vi "DeleteAProperty.vi"(7 "Position Index":T11, 8 "error IO":errorcluster, 10 "JSON Text":string, 11 "Data":T1) -> (0 "error out":errorcluster, 1 "Position Index Out":T11, 2 "JSON Text out":string, 3 "Data Out":T1)   [LabVIEW 2017]
uses:
  <vilib>/JDP Science/JSONtext/JSONtext.lvlib
  8dd03d57-00a7-4a41-af65-d2a72e3468d9.vi
  ab79f004-401f-4e0e-8bc0-55245355768b.vi
  fc2bac9e-75c4-4cb1-9ee7-1f7125c17c3a.vi
  f6ad1758-55d4-4416-b90a-648c1bc133c8.vi
  Ctrl/Property.ctl
  Ctrl/PhysicalChannel.ctl
  Ctrl/Bitfield.ctl
  Ctrl/Register.ctl
  Ctrl/ScaleType.ctl
  Ctrl/Scale.ctl
  Ctrl/EnumValue.ctl
  Ctrl/Enum.ctl
  Ctrl/Caps.ctl
  Ctrl/Data.ctl
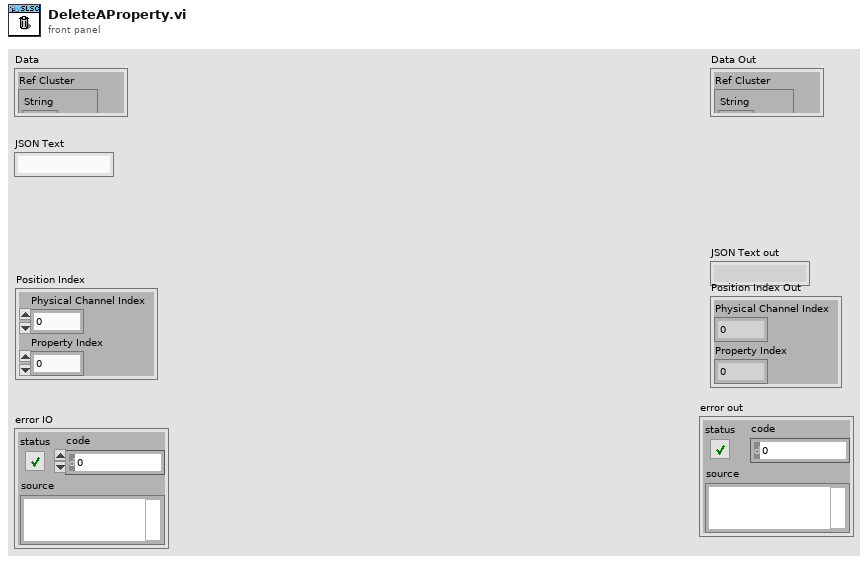
[diagram p1: front panel]
types:
  T1 = typedef "Data.ctl" = cluster{"Ref Cluster":cluster{"String":refnum<vi>, "U8":refnum<vi>, "I8":refnum<vi>, "U32":refnum<vi>, "I32":refnum<vi>, "U64":refnum<vi>, "I64":refnum<vi>, "Ring":refnum<vi>, "DBL":refnum<vi>, "Add":refnum<vi>, "Remove":refnum<vi>, "Property tree":refnum<vi>, "confirm":refnum<vi>}, "JSON Text":string, "Original JSON Text":string, "Caps":T2, "SLSC Output Tree":cluster{"Left Cell String":string, "Child Text":string[], "Child Tag":string, "Item Indent":i32, "Child Only?":bool, "Glyph Index":i32, "offline value":variant}[], "Ref Index and Control Type":cluster{"index":i32, "Datatype":string}, "Selected Type and name":cluster{"Selected Type":enum16{"Property", "Physical Channel", "Other"}, "Selected Property Name":string}, "Update whole Tree?":bool}
  T2 = typedef "Caps.ctl" = cluster{"properties":T3[], "physical channels":T4[], "registers":T5[], "scales":T7[], "enums":T9[], "productName":string}
  T3 = typedef "Property.ctl" = cluster{"name":string, "bitfield":string, "value":variant, "dataType":string, "min":variant, "max":variant, "scale":string, "access":string}
  T4 = typedef "PhysicalChannel.ctl" = cluster{"name":string, "properties":T3[]}
  T5 = typedef "Register.ctl" = cluster{"name":string, "address":i32, "size":i32, "bitfields":T6[], "initialValue":variant, "connectedProperties":string[]}
  T6 = typedef "Bitfield.ctl" = cluster{"name":string, "offset":i32, "size":i32, "signed":bool}
  T7 = typedef "Scale.ctl" = cluster{"name":string, "type":T8, "params":variant}
  T8 = typedef "ScaleType.ctl" = enum16{"NoScale", "Table", "Polynomial", "Linear"}
  T9 = typedef "Enum.ctl" = cluster{"name":string, "values":T10[]}
  T10 = typedef "EnumValue.ctl" = cluster{"name":string, "value":i32}
  T11 = cluster{"Physical Channel Index":i32, "Property Index":i32}
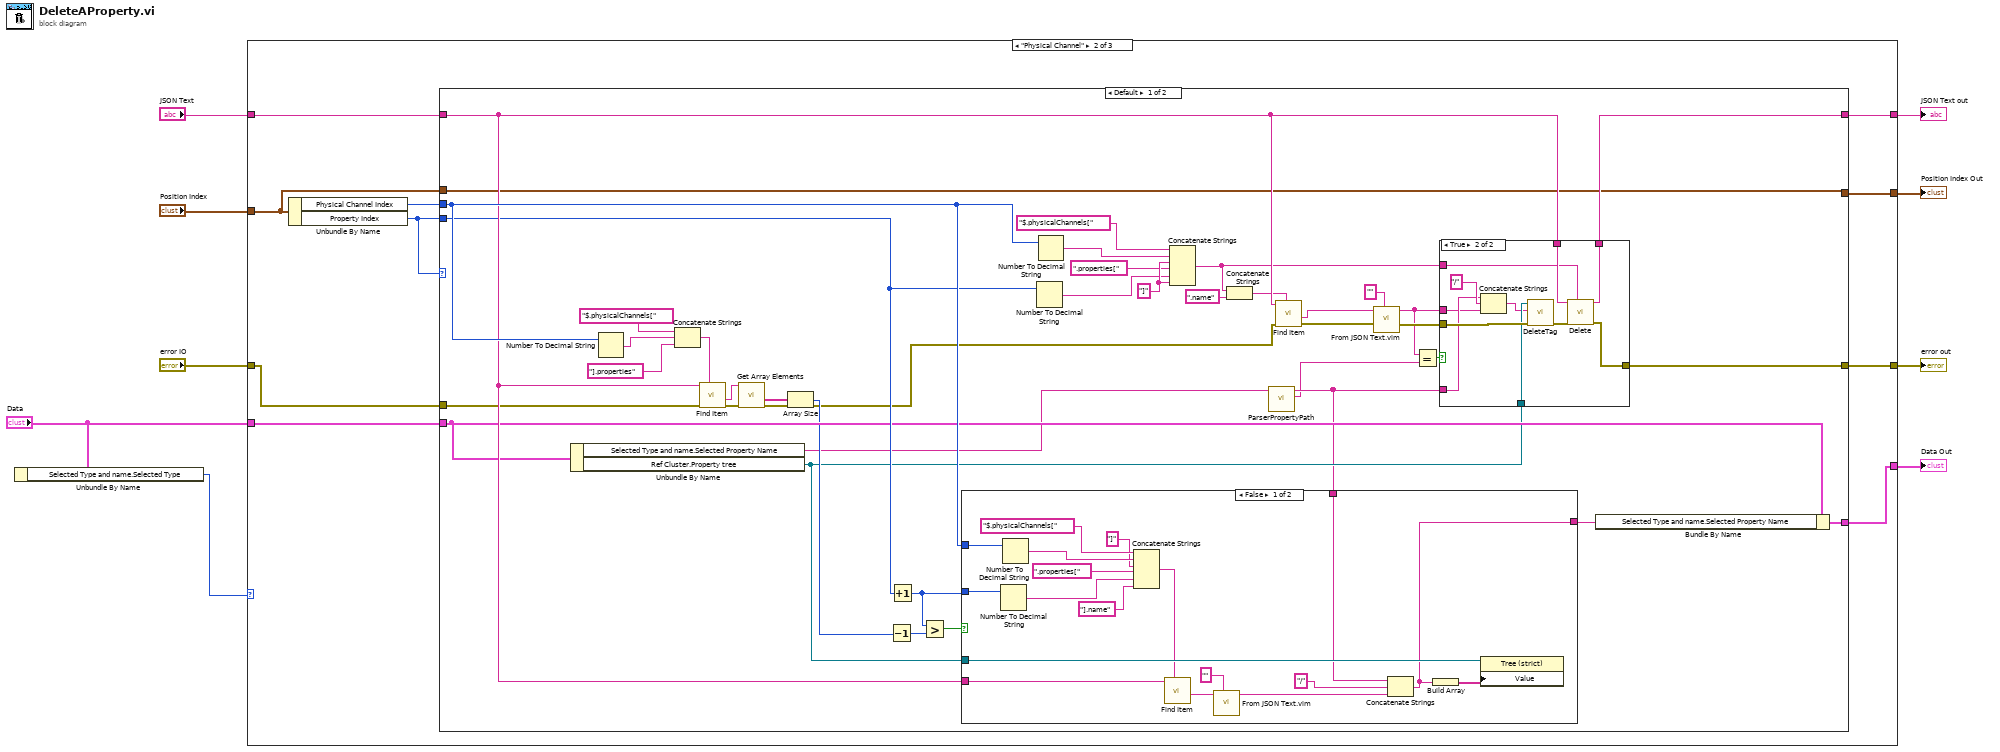
[diagram p0: block diagram]
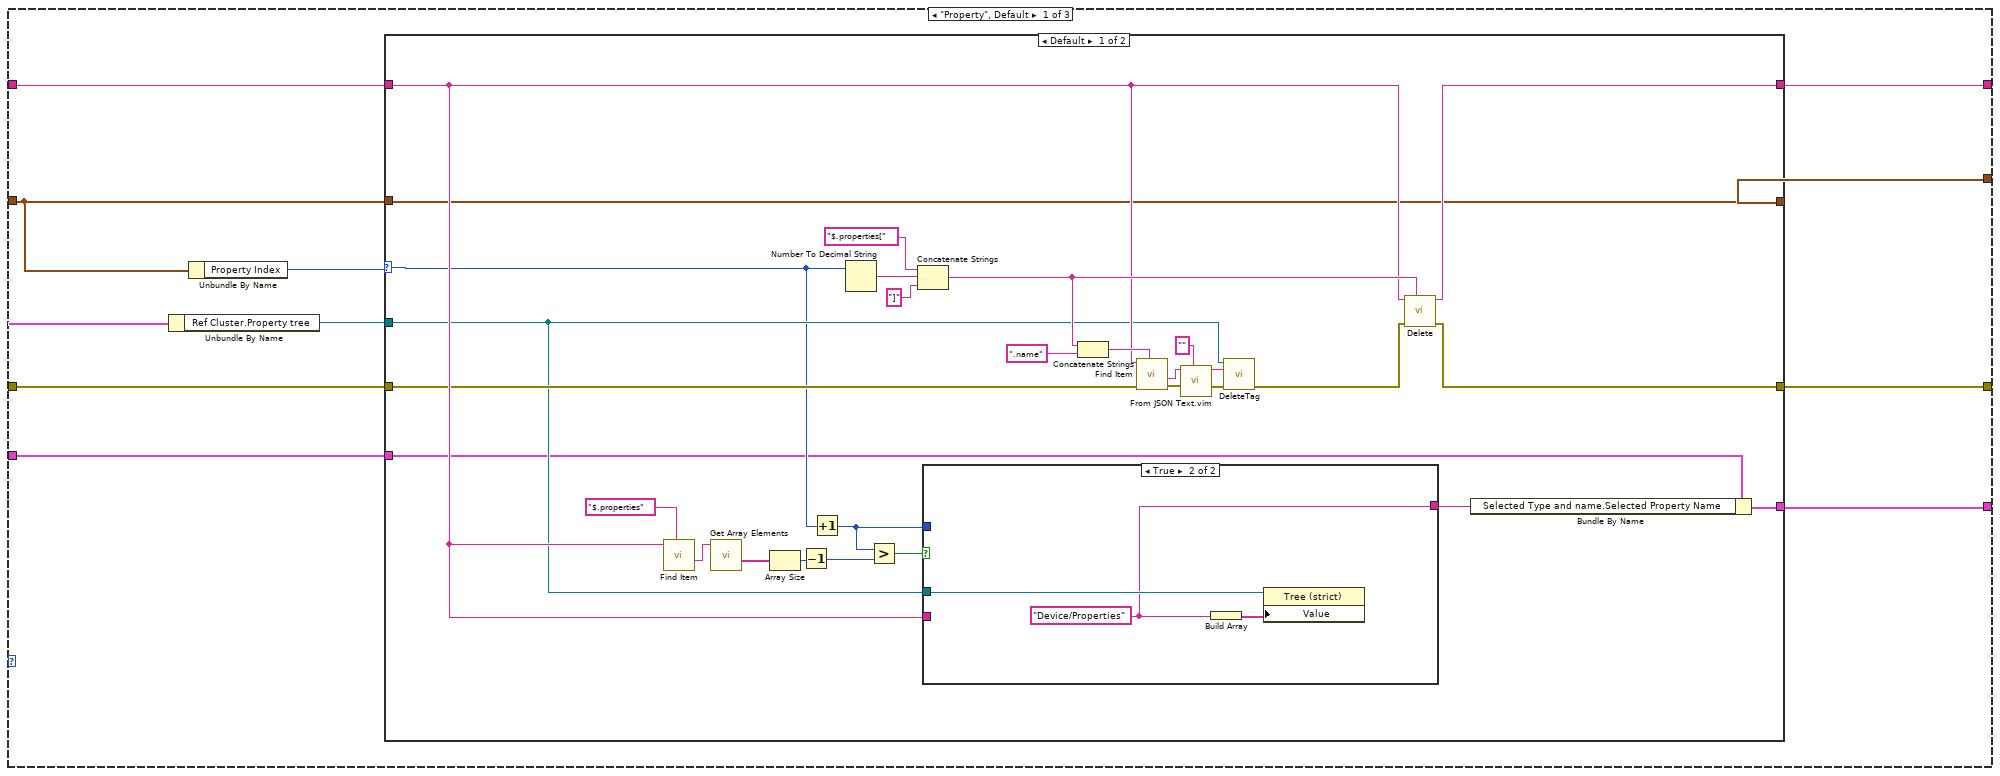
[diagram p2: hidden frame]
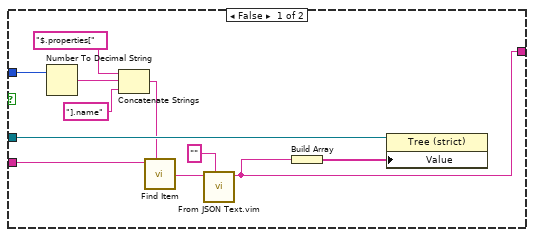
[diagram p3: hidden frame]
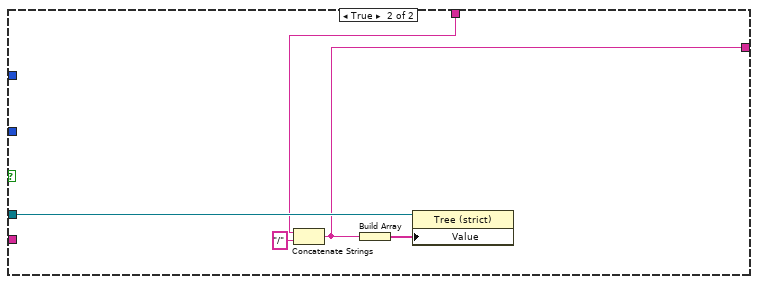
[diagram p6: hidden frame]
diagram:
  n1 = Unbundle By Name("Data") -> ("Selected Type and name.Selected Type"=w1:enum16{"Property", "Physical Channel", "Other"})
  n2 = case shown="\"Physical Channel\"" w1 {
    tunnel: "JSON Text" -> [w17 w73 w160]
    tunnel: "Data" -> [w14 w70 w157]
    tunnel: "error IO" -> [w16 w72 w158]
    tunnel: [w19 w75 w158] -> w4
    tunnel: [w10 w71 w157] -> w3
    tunnel: [w18 w76 w160] -> w6
    tunnel: "Position Index" -> [w13 w67 w159]
    tunnel: [w12 w68 w159] -> w5
    frame "Property", Default {
      n3 = Unbundle By Name(w14) -> ("Ref Cluster.Property tree"=w15:refnum<vi>)
      n4 = Unbundle By Name(w13) -> ("Property Index"=w11:i32)
      n5 = case shown="Default" w11 {
        selector: w11 -> [w23 _]
        tunnel: [w45 w64] -> w19
        tunnel: [w44 w66] -> w18
        tunnel: w17 -> [w28 w66]
        tunnel: w16 -> [w26 w64]
        tunnel: w15 -> [w25 _]
        tunnel: w14 -> [w20 w63]
        tunnel: [w22 w63] -> w10
        tunnel: [w24 w65] -> w12
        tunnel: w13 -> [w24 w65]
        frame Default {
          n6 = call <vilib>:"Find Item.vi"("$Path or Item Name"="$.properties", "JSON"=w28) -> ("<JSON>"=w41:string)  [unwired: 6 in, 3 out]
          n7 = call <vilib>:"Get Array Elements.vi"("JSON"=w41) -> ("<JSON>"=w39:string[])  [unwired: 8 in, 2 out]
          n8 = Array Size(array=w39) -> (size(s)=w38:i32)
          n9 = Decrement(x=w38) -> (x-1=w37:i32)
          n10 = Increment(x=w23) -> (x+1=w42:i32)
          n11 = Number To Decimal String(number=w23) -> (decimal integer string=w48:string)  [unwired: 1 in]
          n12 = Greater?(x=w42, y=w37) -> (0:w43:bool)
          n13 = Concatenate Strings("$.properties[" ("string"), w48, "]" ("string")) -> (w29:string)
          n14 = case shown="True" w43 {
            tunnel: w25 -> [w59 w62]
            tunnel: w28 -> [w52 _]
            tunnel: w42 -> [w51 _]
            tunnel: [w49 w60] -> w21
            frame False {
              n15 = Number To Decimal String(number=w51) -> (decimal integer string=w56:string)  [unwired: 1 in]
              n16 = Concatenate Strings("$.properties[" ("string"), w56, "].name" ("string")) -> (w53:string)
              n17 = call <vilib>:"Find Item.vi"("$Path or Item Name"=w53, "JSON"=w52) -> ("<JSON>"=w58:string)  [unwired: 6 in, 3 out]
              n18 = call "From JSON Text.vim"("Data Type and Default Value"="", "JSON"=w58) -> ("Data out"=w49:string)  [unwired: 8 in, 1 out]
              n19 = Build Array(w49) -> (w50:string[])
              n20 = property class="Tree (strict)"(reference=w59, "Value"=w50) -> ()  [unwired: 1 in, 2 out]
            }
            frame True {
              w60 = "Device/Properties" ("string")
              n21 = Build Array(w60) -> (w61:string[])
              n22 = property class="Tree (strict)"(reference=w62, "Value"=w61) -> ()  [unwired: 1 in, 2 out]
            }
          }
          n23 = Concatenate Strings(w29, ".name" ("string")) -> (w35:string)
          n24 = call <vilib>:"Find Item.vi"("$Path or Item Name"=w35, "error in (no error)"=w26, "JSON"=w28) -> ("error out"=w30:errorcluster, "<JSON>"=w34:string)  [unwired: 5 in, 2 out]
          n25 = call "From JSON Text.vim"("Data Type and Default Value"="", "error in (no error)"=w30, "JSON"=w34) -> ("error out"=w31:errorcluster, "Data out"=w32:string)  [unwired: 7 in]
          n26 = call "DeleteTag.vi"("error in (no error)"=w31, "Specified Item Name"=w32, "Tree reference"=w25) -> ("error out"=w27:errorcluster)  [unwired: 8 in]
          n27 = call <vilib>:"Delete.vi"("$Path or Item Name"=w29, "error in (no error)"=w27, "JSON"=w28) -> ("error out"=w45:errorcluster, "<JSON>"=w44:string)  [unwired: 4 in, 2 out]
          n28 = Bundle By Name(cluster=w20, "Selected Type and name.Selected Property Name"=w21) -> (w22:T1)
        }
        frame -1 {
        }
      }
    }
    frame "Physical Channel" {
      n29 = Unbundle By Name(w67) -> ("Physical Channel Index"=w74:i32, "Property Index"=w69:i32)
      n30 = case shown="Default" w69 {
        tunnel: [w116 w156] -> w76
        tunnel: [w115 w154] -> w75
        tunnel: w74 -> [w114 _]
        tunnel: w73 -> [w113 w156]
        tunnel: w72 -> [w112 w154]
        tunnel: [w111 w153] -> w71
        tunnel: w69 -> [w109 _]
        tunnel: w70 -> [w108 w153]
        tunnel: w67 -> [w80 w155]
        tunnel: [w80 w155] -> w68
        frame Default {
          w105 = "]" ("string")
          n31 = Unbundle By Name(w108) -> ("Selected Type and name.Selected Property Name"=w82:string, "Ref Cluster.Property tree"=w83:refnum<vi>)
          n32 = Number To Decimal String(number=w114) -> (decimal integer string=w97:string)  [unwired: 1 in]
          n33 = Concatenate Strings("$.physicalChannels[" ("$Path or Item Name"), w97, "].properties" ("string")) -> (w95:string)
          n34 = call <vilib>:"Find Item.vi"("$Path or Item Name"=w95, "error in (no error)"=w112, "JSON"=w113) -> ("error out"=w100:errorcluster, "<JSON>"=w101:string)  [unwired: 5 in, 2 out]
          n35 = call <vilib>:"Get Array Elements.vi"("error in (no error)"=w100, "JSON"=w101) -> ("error out"=w84:errorcluster, "<JSON>"=w99:string[])  [unwired: 7 in, 1 out]
          n36 = Array Size(array=w99) -> (size(s)=w93:i32)
          n37 = Decrement(x=w93) -> (x-1=w92:i32)
          n38 = Increment(x=w109) -> (x+1=w94:i32)
          n39 = Greater?(x=w94, y=w92) -> (0:w102:bool)
          n40 = Number To Decimal String(number=w109) -> (decimal integer string=w103:string)  [unwired: 1 in]
          n41 = Number To Decimal String(number=w114) -> (decimal integer string=w106:string)  [unwired: 1 in]
          n42 = Concatenate Strings("$.physicalChannels[" ("$Path or Item Name"), w106, w105, ".properties[" ("string"), w103, w105) -> (w91:string)
          n43 = Concatenate Strings(w91, ".name" ("string")) -> (w89:string)
          n44 = call "ParserPropertyPath.vi"("property"=w82) -> ("name"=w78:string, "pyhsical channel"=w81:string)  [unwired: 7 in]
          n45 = case shown="False" w102 {
            tunnel: w83 -> [w147 w152]
            tunnel: w113 -> [w142 _]
            tunnel: w114 -> [w136 _]
            tunnel: w94 -> [w135 _]
            tunnel: [w131 w149] -> w110
            tunnel: w81 -> [w130 w148]
            frame False {
              n46 = Number To Decimal String(number=w135) -> (decimal integer string=w137:string)  [unwired: 1 in]
              n47 = Number To Decimal String(number=w136) -> (decimal integer string=w140:string)  [unwired: 1 in]
              n48 = Concatenate Strings("$.physicalChannels[" ("$Path or Item Name"), w140, "]", ".properties[" ("string"), w137, "].name" ("string")) -> (w134:string)
              n49 = call <vilib>:"Find Item.vi"("$Path or Item Name"=w134, "JSON"=w142) -> ("<JSON>"=w145:string)  [unwired: 6 in, 3 out]
              n50 = call "From JSON Text.vim"("Data Type and Default Value"="", "JSON"=w145) -> ("Data out"=w143:string)  [unwired: 8 in, 1 out]
              n51 = Concatenate Strings(w130, "/" ("string"), w143) -> (w131:string)
              n52 = Build Array(w131) -> (w146:string[])
              n53 = property class="Tree (strict)"(reference=w147, "Value"=w146) -> ()  [unwired: 1 in, 2 out]
            }
            frame True {
              n54 = Concatenate Strings(w148, "/" ("string")) -> (w149:string)
              n55 = Build Array(w149) -> (w151:string[])
              n56 = property class="Tree (strict)"(reference=w152, "Value"=w151) -> ()  [unwired: 1 in, 2 out]
            }
          }
          n57 = call <vilib>:"Find Item.vi"("$Path or Item Name"=w89, "error in (no error)"=w84, "JSON"=w113) -> ("error out"=w85:errorcluster, "<JSON>"=w88:string)  [unwired: 5 in, 2 out]
          n58 = call "From JSON Text.vim"("Data Type and Default Value"="", "error in (no error)"=w85, "JSON"=w88) -> ("error out"=w86:errorcluster, "Data out"=w79:string)  [unwired: 7 in]
          n59 = Equal?(x=w79, y=w78) -> (x = y?=w77:bool)
          n60 = case shown="True" w77 {
            tunnel: [w118 w129] -> w116
            tunnel: [w117 w128] -> w115
            tunnel: w113 -> [w118 w127]
            tunnel: w91 -> [_ w125]
            tunnel: w86 -> [w117 w124]
            tunnel: w83 -> [_ w123]
            tunnel: w81 -> [_ w120]
            tunnel: w79 -> [_ w119]
            frame False {
            }
            frame True {
              n61 = Concatenate Strings(w120, "/" ("regular expression"), w119) -> (w122:string)
              n62 = call "DeleteTag.vi"("error in (no error)"=w124, "Specified Item Name"=w122, "Tree reference"=w123) -> ("error out"=w126:errorcluster)  [unwired: 8 in]
              n63 = call <vilib>:"Delete.vi"("$Path or Item Name"=w125, "error in (no error)"=w126, "JSON"=w127) -> ("error out"=w128:errorcluster, "<JSON>"=w129:string)  [unwired: 4 in, 2 out]
            }
          }
          n64 = Bundle By Name(cluster=w108, "Selected Type and name.Selected Property Name"=w110) -> (w111:T1)
        }
        frame -1 {
        }
      }
    }
    frame "Other" {
    }
  }
  "JSON Text out" <- w6
  "Position Index Out" <- w5
  "error out" <- w4
  "Data Out" <- w3
